vi "Configure Acquisition.vi"(0 "device session in":refnum<class "Device Session.lvclass">, 1 "pretrigger samples":u64, 2 "number of records is finite (T)":bool=TRUE, 5 "number of records":u64=1, 7 "number of samples":u64=1000, 9 "channels to store":u32[](array[numeric]), 11 "error in":errorcluster, 12 "additional configuration":T1={"record padding (samples)"=0, "require finite records to fit in memory"=TRUE, "timestamps per record"=1, "status fifo depth (records)"=10000}, 13 "channel":u8=1) -> (4 "device session out":refnum<class "Device Session.lvclass">, 6 "actual channels stored":bool[](array[boolean]), 15 "error out":errorcluster)   [LabVIEW 2021, in "Device Session.lvclass"]
doc: "Configures the acquisition. You can specify which channels to acquire from, how many records to acquire, and how many samples to acquire. You must run this VI before running the <B>Initiate</B> VI.\n\n<B>Input Parameters</B>\n\n<B>device session in</B> is a reference to the Device Session object, which contains a session to each instrument design library used in this sample project. This parameter is obtained from the 'Open Session' VI.\n\n<B>number of records is finite (T)</B> specifies whether to acquire a finite number of records, or to acquire records continuously.\n\n<B>pretrigger samples</B> specifies, for every record, the minimum number of samples that must be stored from the time period immediately before the Reference Trigger occurred.\n\n<B>number of records</B> specifies the number of records to acquire. The default value is 1.\n\n<B>number of samples</B> specifies the number of samples to acquire. The default value is 1000.\n\n<B>channels to store</B> specifies the channels to store in memory. By default, only the channels configured using the 'Configure Channel' VI are stored.\n\n<B>additional configuration</B> specifies additional advanced configurations.\n\n<B>additional configuration.record padding (samples)</B> specifies additional padding to allocate for a record. This parameter can be useful in combination with adjusting the Reference Trigger position. The default value is 0.\n\n<B>additional configuration.require finite records to fit in memory</B> specifies that the requested number of records and samples must fit into memory for finite acquisitions. This parameter ensures that requested data cannot be overwritten for finite acquisitions. The default is TRUE.\n\n<B>additional configuration.timestamps per record</B> specifies the number of timestamp values the FPGA captures for each record. This value must match the number of timestamps per record provided to the Write VI of the Multirecord Acquisition FPGA library. The default value is 0.\n\n<B>additional configuration.status fifo depth (records)</B> Sets the depth of the record status DMA FIFO. The Status FIFO reports information about the current state of the acquisition to the host.\nEnsure that the Status FIFO is deep enough for the rate at which the host consumes this FIFO. If the Status FIFO is full, memory writes are delayed. Eventually, this can cause the Write FIFO to fill up and overflow. The host consumes the entire Status FIFO each time you fetch a record or query acquisition status. The value is specified in units of records. The default value is 10,000 records.\n\n<B>error in</B> describes error conditions that occur before this node runs. This input provides standard 'error in' functionality.\n\n<B>Output Parameters</B>\n\n<B>device session out</B> passes a reference to the session to the next VI.\n\n<B>actual channels stored</B> returns the number of channels stored as a power of two.\n\n<B>error out</B> contains error information. This output provides standard 'error out' functionality."
uses:
  Device Session.lvclass
  <instrlib>/_niInstr/Multirecord Acquisition/Interface/v1/Host/Public/Additional Acquisition Configuration.ctl
  Device Session.lvclass/Device Session.ctl
  <vilib>/Utility/error.llb/Error Cluster From Error Code.vi
  <vilib>/rvi/errors/niLvFpgaAdjustHostInterfaceError.vi
  <vilib>/rvi/interface/nirviReadWriteControl/nirviReadWriteControl.xnode
  FPGA Refnum.ctl
  <instrlib>/_niInstr/Multirecord Acquisition/Interface/v1/Host/niInstr Multirecord Acquisition v1 Host.lvclass
  <vilib>/rvi/interface/Simulation/niFpgaSimulationCallBeginRW.vi
  NiFpgaLv.dll
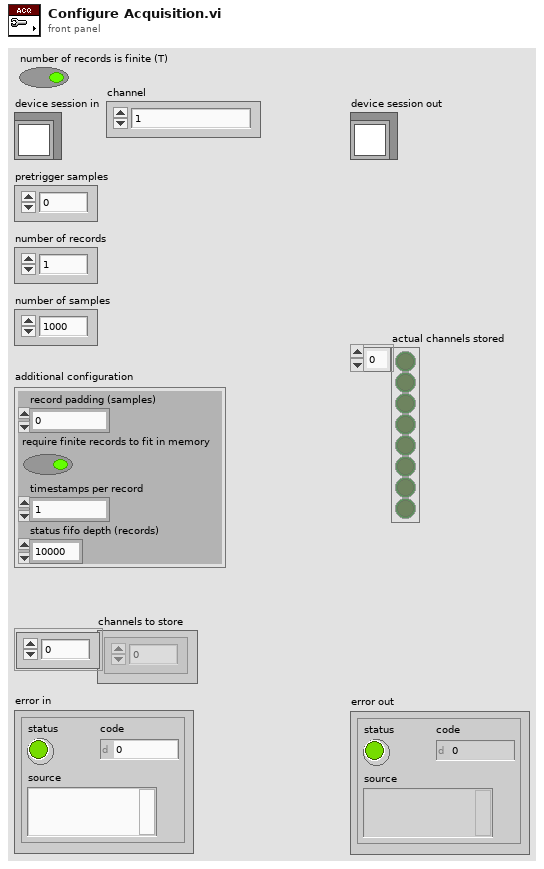
[diagram p1: front panel]
types:
  T1 = typedef "niInstr Multirecord Acquisition v1 Host.lvclass/Additional Acquisition Configuration.ctl" = cluster{"record padding (samples)":u64, "require finite records to fit in memory":bool, "timestamps per record":u32, "status fifo depth (records)":u32}
  T2 = typedef "Device Session.lvclass/Device Session Object.ctl" = cluster{"fpga reference":T3, "reg bus":refnum<class "niInstr FIFO Register Bus v1 Host.lvclass">, "subsystem map":refnum<class "niInstr Subsystem Map v1 Host.lvclass">, "cal data":refnum<class "niHSAI Cal Data v1 Host.lvclass">, "config":refnum<class "niHSAI Group A Config v1 Host.lvclass">, "acquisition refs":refnum<class "niInstr Multirecord Acquisition v1 Host.lvclass">[], "acquisition 1":refnum<class "niInstr Multirecord Acquisition v1 Host.lvclass">, "number of selected acq channels":u8, "selected acq channels":bool[], "number of channels":u32, "configured channels":bool[], "acq configuration":cluster{"number of samples":u64, "number of records":u64, "pretrigger samples":u64}, "actual channel configuration":T4[], "sample clock rate (Hz)":dbl, "scaling coefficients":T8[]}
  T3 = typedef "Device Session.lvclass/FPGA Refnum.ctl" = refnum<k20>
  T4 = typedef "niHSAI Types v1 Host.lvlib/Channel Configuration.ctl" = cluster{"channel":u32, "coupling":T5, "impedance":T6, "bandwidth":T7, "vertical range":dbl, "vertical offset":dbl}
  T5 = typedef "niHSAI Types v1 Host.lvlib/Coupling.ctl" = enum8{"Default", "DC", "AC"}
  T6 = typedef "niHSAI Types v1 Host.lvlib/Impedance.ctl" = enum8{"Default", "1 mega ohm", "50 ohm"}
  T7 = typedef "niHSAI Types v1 Host.lvlib/Bandwidth.ctl" = enum8{"Default", "Full Bandwidth", "Anti-alias Filter", "150 MHz"}
  T8 = typedef "niInstr Multirecord Acquisition v1 Host.lvclass/Scaling Coefficient.ctl" = cluster{"gain":dbl, "offset":dbl}
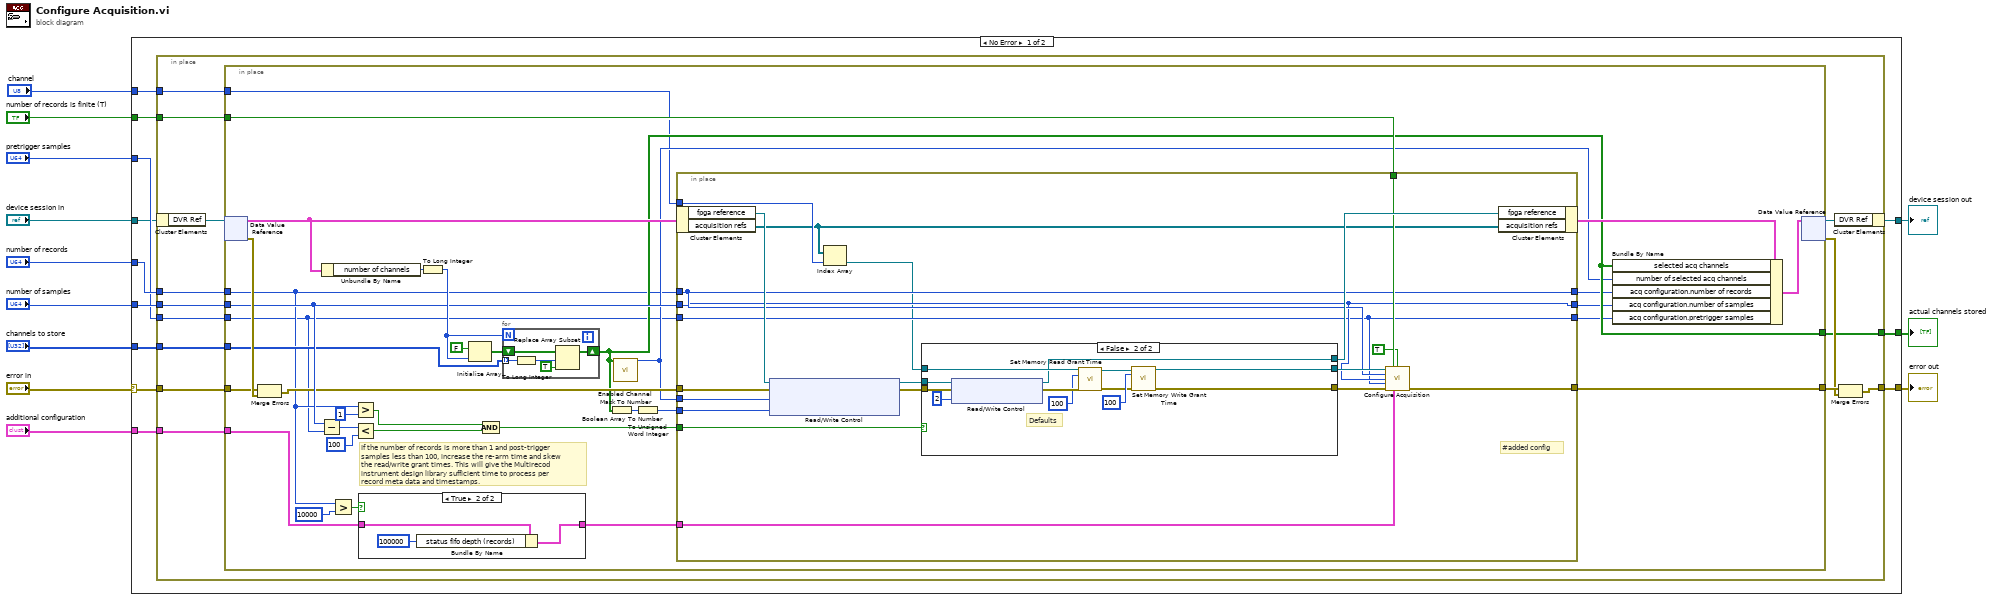
[diagram p0: block diagram]
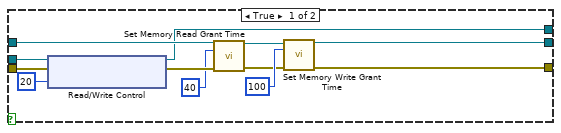
[diagram p2: hidden frame]
diagram:
  n1 = case shown="No Error" "error in" {
    selector: "error in" -> [w24 w127]
    tunnel: [w16 w127] -> w11
    tunnel: "device session in" -> [w14 w126]
    tunnel: [w15 w126] -> w9
    tunnel: "number of records" -> [w23 _]
    tunnel: "number of samples" -> [w22 _]
    tunnel: "channels to store" -> [w21 _]
    tunnel: [w20 _] -> w5
    tunnel: "pretrigger samples" -> [w19 _]
    tunnel: "additional configuration" -> [w18 _]
    tunnel: "number of records is finite (T)" -> [w17 _]
    tunnel: "channel" -> [w13 _]
    frame No Error {
      n2 = in-place {
        in-place-border: w24 -> [w38]
        in-place-border: w23 -> [w37]
        in-place-border: w22 -> [w36]
        in-place-border: w21 -> [w33]
        in-place-border: [w32] -> w20
        in-place-border: w19 -> [w31]
        in-place-border: w18 -> [w30]
        in-place-border: w17 -> [w29]
        in-place-border: [w28] -> w16
        in-place-border: w13 -> [w25]
        n3 = in-place-cluster #1(w14) -> ("DVR Ref"=w27:refnum<data-value>)
        n4 = in-place {
          in-place-border: w38 -> [w67]
          in-place-border: [w70] -> w35
          in-place-border: w37 -> [w41]
          in-place-border: w36 -> [w53]
          in-place-border: w33 -> [w42]
          in-place-border: [w47] -> w32
          in-place-border: w31 -> [w40]
          in-place-border: w30 -> [w51]
          in-place-border: w29 -> [w64]
          in-place-border: w25 -> [w39]
          # "If the number of records is more than 1 and post-trigger samples less than 100, increase the re-arm time and skew the read/write grant times. This will give the Multirecod instrument design library sufficient time to process per record meta data and timestamps."
          n5 = in-place-dvr #2(w27) -> (w49:T2, w71:errorcluster)
          n6 = Merge Errors(w67, w71) -> (w52:errorcluster)
          n7 = Subtract(x=w53, y=w40) -> (x-y=w61:u64)
          n8 = Unbundle By Name(w49) -> ("number of channels"=w63:u32)
          n9 = Greater?(x=w41, y=u64 10000) -> (0:w54:bool)
          n10 = Greater?(x=w41, y=u64 1) -> (0:w58:bool)
          n11 = Less?(x=w61, y=u64 100) -> (x < y?=w57:bool)
          n12 = case shown="True" w54 {
            tunnel: w51 -> [w117 w120]
            tunnel: [w117 w118] -> w50
            frame False {
            }
            frame True {
              n13 = Bundle By Name(cluster=w120, "status fifo depth (records)"=u32 100000) -> (w118:T1)
            }
          }
          n14 = To Long Integer(number=w63) -> (32bit integer=w62:i32)
          n15 = Initialize Array(FALSE, w62) -> (w65:bool[])
          n16 = And(x=w58, y=w57) -> (x .and. y?=w56:bool)
          n17 = for {
            N: w62 -> [_]
            tunnel: w42 -> [w122] mode=indexing
            shift-right: [w124] -> w47
            shift-left: w65 -> [w123]
            n18 = To Long Integer(number=w122) -> (32bit integer=w121:i32)
            n19 = Replace Array Subset(array=w123, new element=TRUE ("new element/subarray"), index=w121) -> (w124:bool[])
          }
          n20 = Boolean Array To Number(Boolean array=w47) -> (number=w69:u32)
          n21 = call "Enabled Channel Mask To Number.vi"("selected acquisition channels to store"=w47) -> ("number of selected channels"=w46:u8)  [unwired: 14 in]
          n22 = To Unsigned Word Integer(number=w69) -> (unsigned 16bit integer=w68:u16)
          n23 = in-place {
            in-place-border: [w80] -> w70
            in-place-border: w68 -> [w92]
            in-place-border: w64 -> [w82]
            in-place-border: w56 -> [w87]
            in-place-border: w40 -> [w77]
            in-place-border: w53 -> [w78]
            in-place-border: w52 -> [w86]
            in-place-border: w41 -> [w79]
            in-place-border: w46 -> [w85]
            in-place-border: w50 -> [w76]
            in-place-border: [w79] -> w45
            in-place-border: [w78] -> w44
            in-place-border: [w77] -> w43
            in-place-border: w39 -> [w75]
            # "#added config"
            n24 = in-place-cluster #3(w49) -> ("fpga reference"=w84:T3, "acquisition refs"=w73:refnum<class "niInstr Multirecord Acquisition v1 Host.lvclass">[])
            n25 = xnode "Read/Write Control"("FPGA VI Reference In"=w84, "error in"=w86, "channel.number of channels"=w85, "channel.enable mask"=w92) -> ("FPGA VI Reference Out"=w91:T3, "error out"=w90:errorcluster)
            n26 = Index Array(array=w73, index=w75) -> (element=w74:refnum<class "niInstr Multirecord Acquisition v1 Host.lvclass">)
            n27 = case shown="False" w87 {
              tunnel: w74 -> [w98 w110]
              tunnel: w91 -> [w99 w111]
              tunnel: w90 -> [w97 w109]
              tunnel: [w94 w105] -> w89
              tunnel: [w96 w108] -> w88
              tunnel: [w93 w106] -> w83
              frame True {
                n28 = xnode "Read/Write Control"("FPGA VI Reference In"=w99, "error in"=w97, "trigger.rearm delay"=u16 20 ("trigger.rearm time")) -> ("FPGA VI Reference Out"=w93:T3, "error out"=w104:errorcluster)
                n29 = call-dynamic "Set Memory Read Grant Time.vi"("session in"=w98, "grant time (clocks)"=u32 40, "error in"=w104) -> ("session out"=w100:refnum<class "niInstr Multirecord Acquisition v1 Host.lvclass">, "error out"=w101:errorcluster)  [unwired: 11 in]
                n30 = call-dynamic "Set Memory Write Grant Time.vi"("session in"=w100, "grant time (clocks)"=u32 100, "error in"=w101) -> ("session out"=w96:refnum<class "niInstr Multirecord Acquisition v1 Host.lvclass">, "error out"=w94:errorcluster)  [unwired: 11 in]
              }
              frame False {
                # "Defaults"
                n31 = xnode "Read/Write Control"("FPGA VI Reference In"=w111, "error in"=w109, "trigger.rearm delay"=u16 2 ("trigger.rearm time")) -> ("FPGA VI Reference Out"=w106:T3, "error out"=w116:errorcluster)
                n32 = call-dynamic "Set Memory Read Grant Time.vi"("session in"=w110, "grant time (clocks)"=u32 100, "error in"=w116) -> ("session out"=w112:refnum<class "niInstr Multirecord Acquisition v1 Host.lvclass">, "error out"=w113:errorcluster)  [unwired: 11 in]
                n33 = call-dynamic "Set Memory Write Grant Time.vi"("session in"=w112, "grant time (clocks)"=u32 100, "error in"=w113) -> ("session out"=w108:refnum<class "niInstr Multirecord Acquisition v1 Host.lvclass">, "error out"=w105:errorcluster)  [unwired: 11 in]
              }
            }
            n34 = call-dynamic "Configure Acquisition.vi"("session in"=w88, "number of records is finite"=w82, "number of samples is finite"=TRUE, "number of records"=w79, "number of samples"=w78, "pretrigger samples"=w77, "error in"=w89, "additional acquisition configuration"=w76) -> ("error out"=w80:errorcluster)  [unwired: 5 in, 2 out]
            n35 = in-place-cluster #3("fpga reference"=w83, "acquisition refs"=w73) -> (w48:T2)
          }
          n36 = Bundle By Name(cluster=w48, "selected acq channels"=w47, "number of selected acq channels"=w46, "acq configuration.number of records"=w45, "acq configuration.number of samples"=w44, "acq configuration.pretrigger samples"=w43) -> (w72:T2)
          n37 = in-place-dvr #2(w72) -> (w26:refnum<data-value>, w34:errorcluster)
        }
        n38 = in-place-cluster #1("DVR Ref"=w26) -> (w15:refnum<class "Device Session.lvclass">)
        n39 = Merge Errors(w35, w34) -> (w28:errorcluster)
      }
    }
    frame Error {
    }
  }
  "error out" <- w11
  "device session out" <- w9
  "actual channels stored" <- w5
